vi "decodeNil.vi"(8 "error in (no error)":errorcluster, 10 "ByteArray":u8[](array[numeric])) -> (0 "error out":errorcluster, 2 "variant":variant, 3 "RemainingBytes":u8[](array[numeric]), 5 "Type":string)   [LabVIEW 2020, in "MsgPack.lvlib"]
uses:
  MsgPack.lvlib
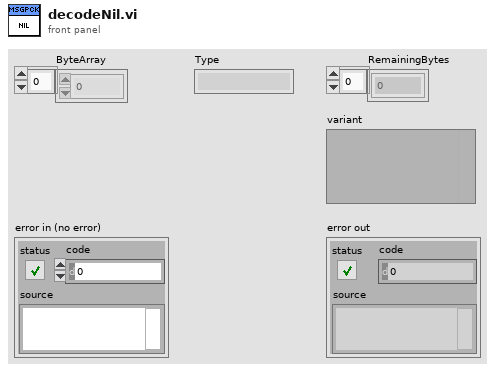
[diagram p1: front panel]
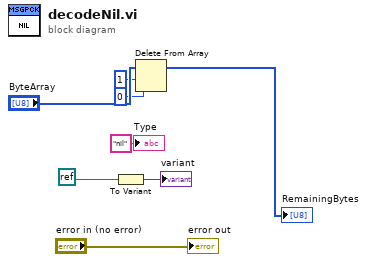
[diagram p0: block diagram]
diagram:
  n1 = To Variant(anything=refnum<k0> refnum) -> (Variant=→"variant":variant)
  n2 = Delete From Array(array="ByteArray", length=1, index=0) -> (array with subset deleted=→"RemainingBytes":u8[])  [unwired: 1 out]
  "error out" <- "error in (no error)"
  "Type" <- "nil"
